vi "select_sample_for_c_parameter.vi"(8 "Error In":errorcluster, 10 "Sample":string, 11 "File Path":path) -> (0 "Error Out":errorcluster, 1 "Xi":T2, 2 "Selected Sample":string, 3 "selected path":path)   [LabVIEW 2019]
doc: "Get the user to select a data directory, sample name, and sequence to use for determining the c-parameter."
uses:
  xi_angles_enum_typedef.ctl
  select_sample_states_enum_typedef.ctl
panel:
  out "45 sequence":T1(plugin-control)
  out "0 sequence":T1(plugin-control)
  in  "45 Degree":bool
  in  "0 Degree":bool
  # "Select Sequence"
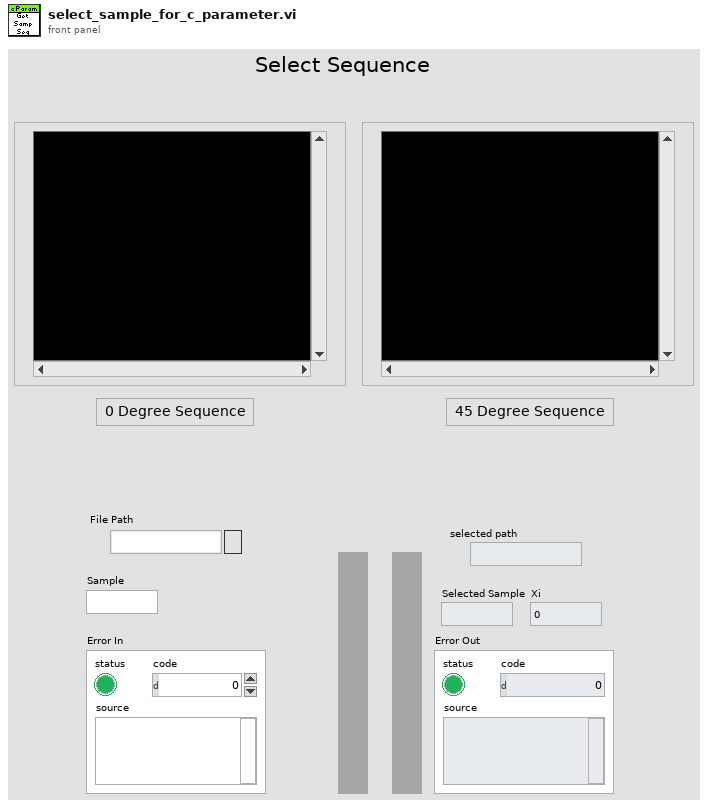
[diagram p1: front panel]
types:
  T1 = typedef "IMAQ Image.ctl" = refnum<image>
  T2 = typedef "xi_angles_enum_typedef.ctl" = enum16{"0", "45"}
  T3 = typedef "select_sample_states_enum_typedef.ctl" = enum16{"Wait", "Set Sequence 45", "Set Sequence 0", "Shutdown", "Load", "Initialize"}
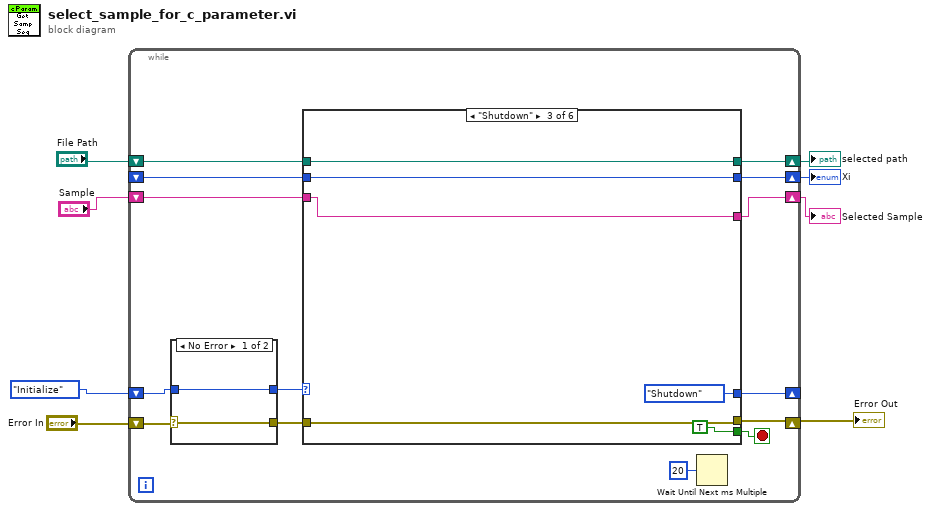
[diagram p0: block diagram]
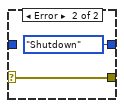
[diagram p2: hidden frame]
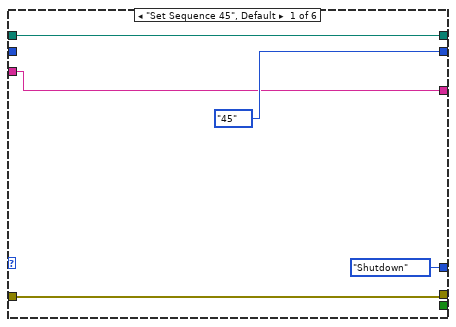
[diagram p3: hidden frame]
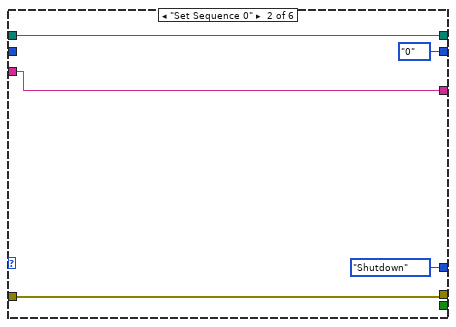
[diagram p4: hidden frame]
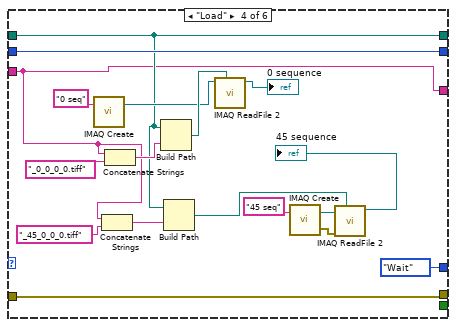
[diagram p5: hidden frame]
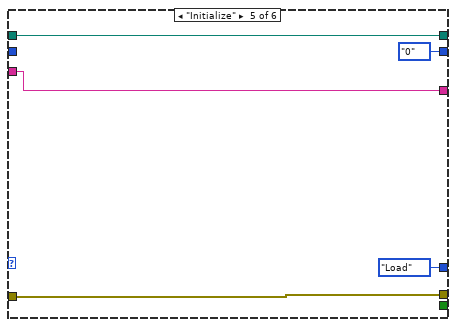
[diagram p6: hidden frame]
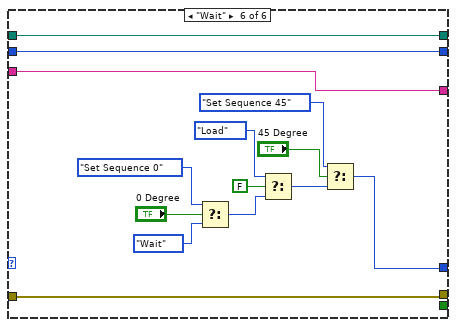
[diagram p7: hidden frame]
diagram:
  n1 = while {
    shift-right: [w17] -> w3
    shift-left: "File Path" -> [w15]
    shift-right: [w16] -> w4
    shift-left: _ -> [w14]
    shift-right: [w13] -> _
    shift-left: select_sample_states_enum_typedef."Initialize" -> [w20]
    shift-right: [w18] -> w6
    shift-left: "Error In" -> [w22]
    shift-right: [w10] -> w5
    shift-left: "Sample" -> [w9]
    stop <- w12 stop-if-true
    n2 = case shown="No Error" w22 {
      selector: w22 -> [w24 w26]
      tunnel: [w24 w26] -> w21
      tunnel: w20 -> [w23 _]
      tunnel: [w23 select_sample_states_enum_typedef."Shutdown"] -> w19
      frame No Error {
      }
      frame Error {
      }
    }
    n3 = case shown="\"Shutdown\"" w19 {
      tunnel: w21 -> [w28 w33 w39 w58 w63 w68]
      tunnel: [w28 w33 w39 w58 w63 w68] -> w18
      tunnel: [w30 w35 w41 w45 w62 w79] -> w17
      tunnel: [xi_angles_enum_typedef."45" ("Xi") xi_angles_enum_typedef."0" ("Xi") w42 w59 xi_angles_enum_typedef."0" ("Xi") w78] -> w16
      tunnel: w15 -> [w30 w35 w41 w45 w62 w79]
      tunnel: w14 -> [_ _ w42 w59 _ w78]
      tunnel: [select_sample_states_enum_typedef."Shutdown" select_sample_states_enum_typedef."Shutdown" select_sample_states_enum_typedef."Shutdown" select_sample_states_enum_typedef."Wait" select_sample_states_enum_typedef."Load" w69] -> w13
      tunnel: [_ _ TRUE _ _ _] -> w12
      tunnel: [w27 w32 w37 w43 w61 w66] -> w10
      tunnel: w9 -> [w27 w32 w37 w43 w61 w66]
      frame "Set Sequence 45", Default {
      }
      frame "Set Sequence 0" {
      }
      frame "Shutdown" {
      }
      frame "Load" {
        n4 = call "IMAQ Create"("Image Name"="0 seq") -> ("New Image"=w53:T1)  [unwired: 4 in, 1 out]
        n5 = Concatenate Strings(w43, "_45_0_0_0.tiff" ("string")) -> (w46:string)
        n6 = Concatenate Strings(w43, "_0_0_0_0.tiff" ("string")) -> (w56:string)
        n7 = Build Path(base path=w45, name or relative path=w56) -> (appended path=w55:path)
        n8 = Build Path(base path=w45, name or relative path=w46) -> (appended path=w44:path)
        n9 = call "IMAQ ReadFile 2"("File Path"=w55, "Image"=w53) -> ("Image Out"=→"0 sequence":T1)  [unwired: 5 in, 4 out]
        n10 = call "IMAQ Create"("Image Name"="45 seq") -> ("New Image"=w49:T1, "error out"=w50:errorcluster)  [unwired: 4 in]
        n11 = call "IMAQ ReadFile 2"("File Path"=w44, "error in (no error)"=w50, "Image"=w49) -> ("Image Out"=→"45 sequence":T1)  [unwired: 4 in, 4 out]
      }
      frame "Initialize" {
      }
      frame "Wait" {
        n12 = Select(t=select_sample_states_enum_typedef."Set Sequence 0", s="0 Degree", f=select_sample_states_enum_typedef."Wait") -> (s? t:f=w74:T3)
        n13 = Select(t=select_sample_states_enum_typedef."Load", s=FALSE, f=w74) -> (s? t:f=w71:T3)
        n14 = Select(t=select_sample_states_enum_typedef."Set Sequence 45", s="45 Degree", f=w71) -> (s? t:f=w69:T3)
      }
    }
    n15 = Wait Until Next ms Multiple(millisecond multiple=u32 20) -> ()  [unwired: 1 out]
  }
  "Error Out" <- w6
  "Selected Sample" <- w5
  "Xi" <- w4
  "selected path" <- w3
